vi "F Dwf Analog Out Limitation Get.vi"(8 "error in (no error)":errorcluster, 9 "plimit":dbl, 10 "idxChannel":i32, 11 "hdwf":i32) -> (0 "error out":errorcluster, 1 "plimit out":dbl, 3 "function return":i32)   [LabVIEW 2019, in "Olasdwf.lvlib"]
doc: "DWFAPI int FDwfAnalogOutLimitationGet(HDWF hdwf, int idxChannel, double *plimit);"
uses:
  Olasdwf.lvlib
  Windows/System32/dwf.dll
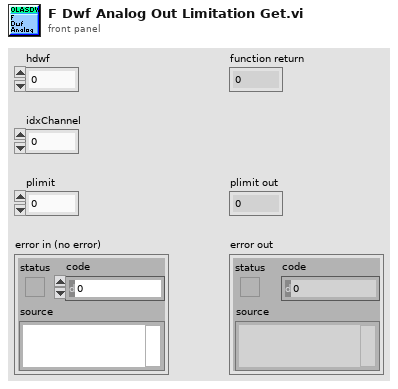
[diagram p1: front panel]
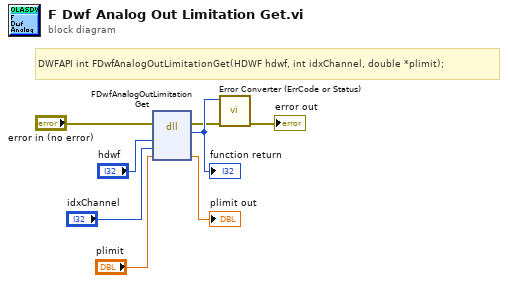
[diagram p0: block diagram]
diagram:
  # "DWFAPI int FDwfAnalogOutLimitationGet(HDWF hdwf, int idxChannel, double *plimit);"
  n1 = dll-call lib="C:/Windows/System32/dwf.*" fn="FDwfAnalogOutLimitationGet"(error in="error in (no error)", "hdwf"="hdwf", "idxChannel"="idxChannel", "plimit"="plimit") -> (error out=w2:errorcluster, w8:i32, "plimit"=→"plimit out":dbl)  [unwired: 4 in, 1 out]
  "function return" <- w8
  n2 = call "Error Converter (ErrCode or Status).vi"("error in (no error)"=w2, "error code"=w8) -> ("error out"=→"error out":errorcluster)  [unwired: 9 in]
